vi "sub_psk_symbol_map_gen.vi"(9 "Gray code?":bool=TRUE, 11 "M-PSK":i32=4) -> (1 "index map":u32[](array[numeric]), 3 "symbol map":cdb[](array[numeric]))   [LabVIEW 2014]
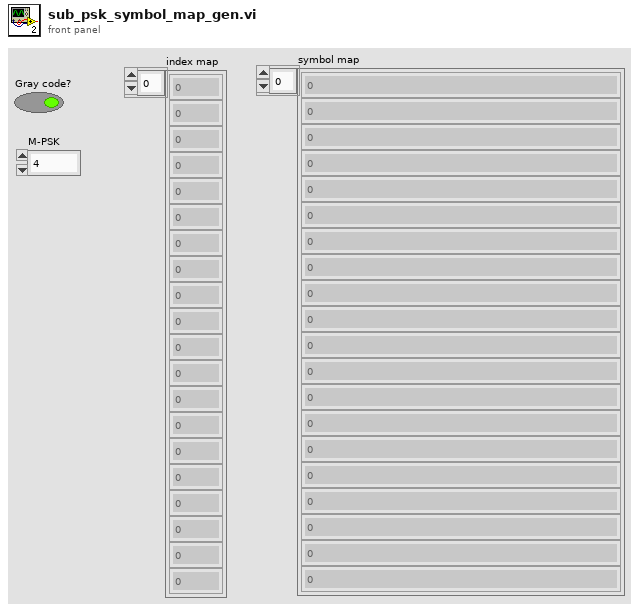
[diagram p1: front panel]
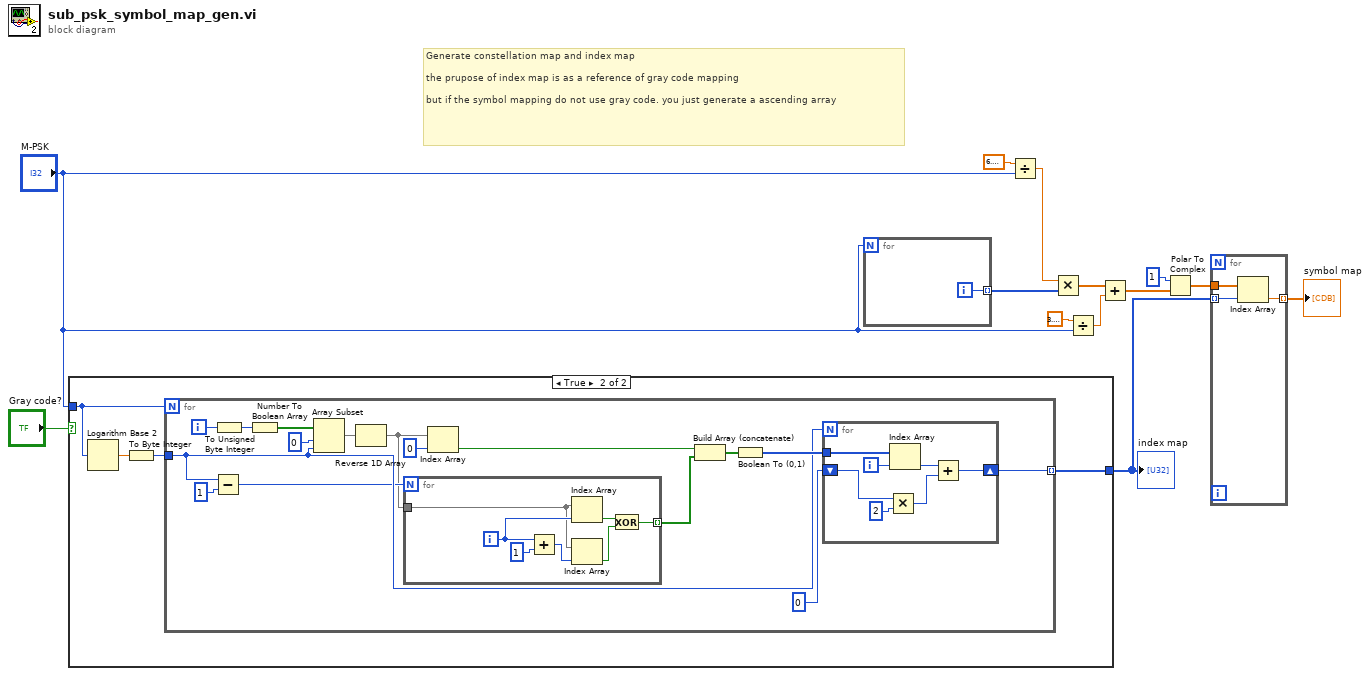
[diagram p0: block diagram]
diagram:
  # "Generate constellation map and index map\n\nthe prupose of index map is as a reference of gray code mapping\n\nbut if the symbol mapping do not use gray code. you just generate a ascending array"
  n1 = case shown="True" "Gray code?" {
    tunnel: "M-PSK" -> [w15 w19]
    tunnel: [w14 w17] -> w3
    frame False {
      n2 = for {
        N: w15 -> [_]
        tunnel: [w16] -> w14 mode=indexing
        i -> [w16]
      }
    }
    frame True {
      n3 = Logarithm Base 2(1:w19) -> (0:w20:dbl)
      n4 = To Byte Integer(number=w20) -> (8bit integer=w18:i8)
      n5 = for {
        N: w19 -> [_]
        tunnel: w18 -> [w29]
        tunnel: [w30] -> w17 mode=indexing
        i -> [w36]
        n6 = Subtract(x=w29, y=1) -> (x-y=w27:i32)
        n7 = To Unsigned Byte Integer(number=w36) -> (unsigned 8bit integer=w35:u8)
        n8 = Number To Boolean Array(number=w35) -> (Boolean array=w33:bool[])
        n9 = Array Subset(array=w33, index=0, length=w29) -> (w23:bool[])
        n10 = Reverse 1D Array(array=w23) -> (reversed array=w22:bool[])
        n11 = for {
          N: w27 -> [_]
          tunnel: [w37] -> w25 mode=indexing
          tunnel: w22 -> [w39]
          i -> [w40]
          n12 = Add(x=w40, y=1) -> (x+y=w43:i32)
          n13 = Index Array(array=w39, index=w40) -> (element=w38:bool)
          n14 = Index Array(array=w39, index=w43) -> (element=w41:bool)
          n15 = Exclusive Or(1:w41, 2:w38) -> (0:w37:bool)
        }
        n16 = Index Array(array=w22, index=0) -> (element=w26:bool)
        n17 = Build Array (concatenate)(w26, w25) -> (w24:bool[])
        n18 = Boolean To (0,1)(Boolean=w24) -> (0, 1=w32:i16[])
        n19 = for {
          N: w29 -> [_]
          tunnel: w32 -> [w50]
          shift-right: [w45] -> w30
          shift-left: 0 -> [w46]
          i -> [w44]
          n20 = Multiply(x=w46, y=2) -> (x*y=w47:i32)
          n21 = Index Array(array=w50, index=w44) -> (element=w48:i16)
          n22 = Add(x=w48, y=w47) -> (x+y=w45:i32)
        }
      }
    }
  }
  "index map" <- w3
  n23 = for {
    N: "M-PSK" -> [_]
    tunnel: [w51] -> w10 mode=indexing
    i -> [w51]
  }
  n24 = Divide(x=6.283185307179586, y="M-PSK") -> (x/y=w11:dbl)
  n25 = Multiply(x=w11, y=w10) -> (x*y=w8:dbl[])
  n26 = Divide(x=3.141592653589793, y="M-PSK") -> (x/y=w4:dbl)
  n27 = Add(x=w8, y=w4) -> (x+y=w7:dbl[])
  n28 = Polar To Complex(1:w7, 2:1) -> (0:w2:cdb[])
  n29 = for {
    tunnel: w3 -> [w54] mode=indexing
    tunnel: w2 -> [w53]
    tunnel: [w52] -> w1 mode=indexing
    n30 = Index Array(array=w53, index=w54) -> (element=w52:cdb)
  }
  "symbol map" <- w1
